vi "measVoltGlobVars.vi"() -> ()   [LabVIEW 2014]
panel:
  out "timedOutWhileHandshake":bool
  in  "measVoltTimeout(25ns)":i32
  in  "measVoltPulseLength(25ns)":i32
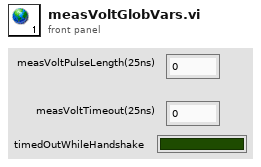
[diagram p1: front panel]
diagram:
